vi "数字量输出自动检测_fast.vi"(11 "测试值":enum16{"0", "1"}(ring)) -> ()   [LabVIEW 2010]
uses:
  全局量/试验配置信息.vi
panel:
  in  "CAN端口":u16
  out "结束？":bool
  in  "同步_2":i32
  in  "同步_1":i32
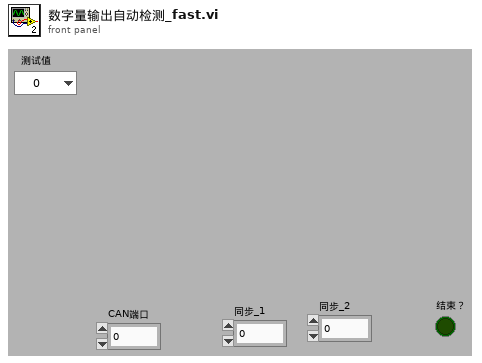
[diagram p1: front panel]
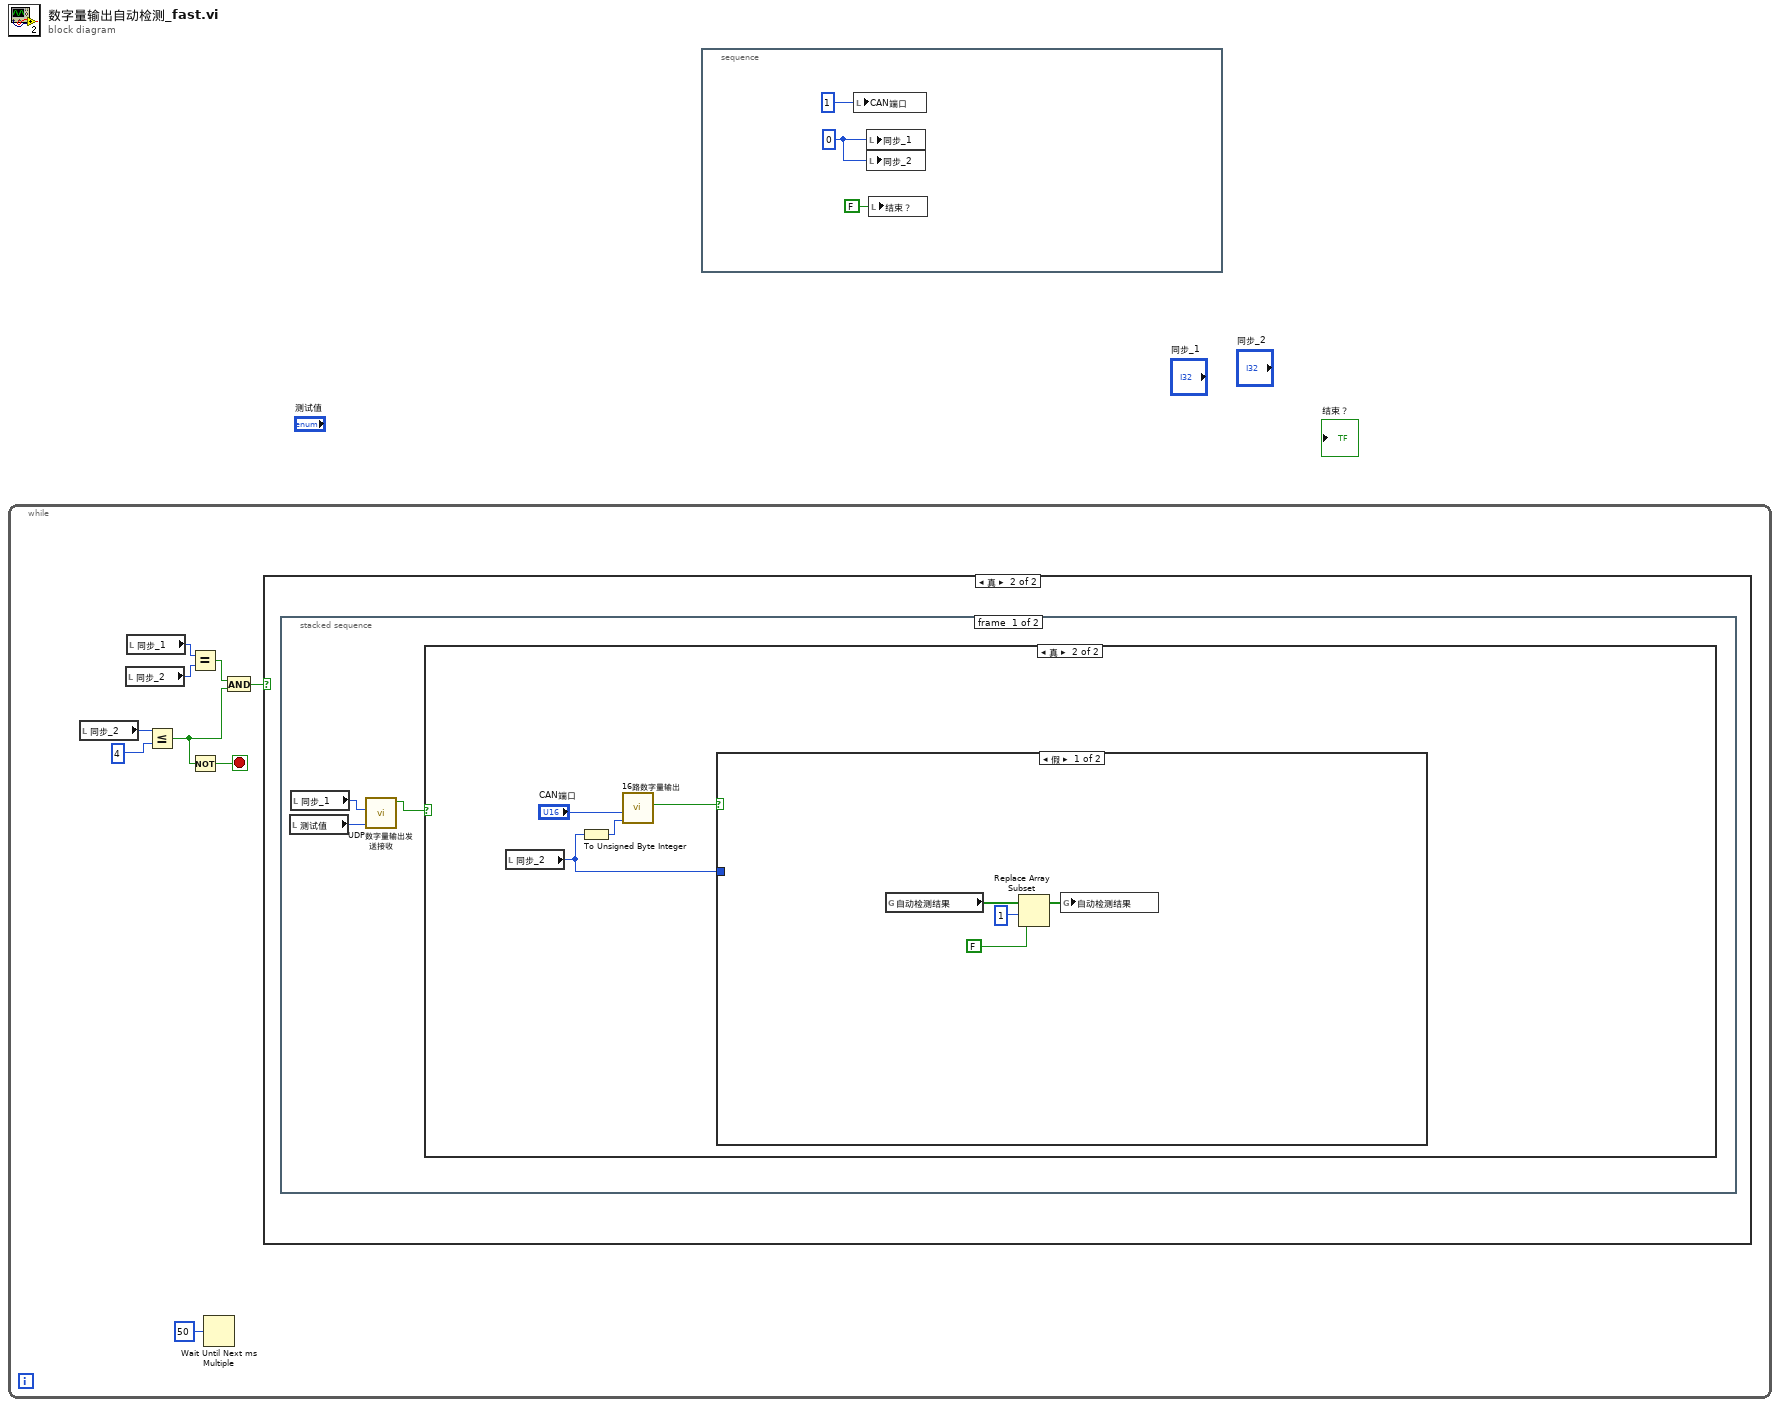
[diagram p0: block diagram]
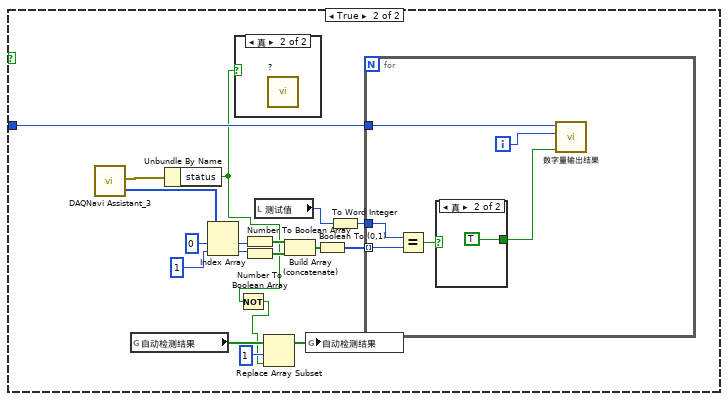
[diagram p4: hidden frame]
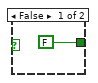
[diagram p6: hidden frame]
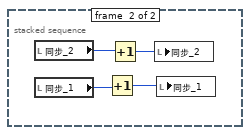
[diagram p7: hidden frame]
diagram:
  n1 = while {
    stop <- w4 stop-if-true
    n2 = local read "同步_2"() -> (w2:i32)
    n3 = local read "同步_2"() -> (w7:i32)
    n4 = local read "同步_1"() -> (w8:i32)
    n5 = Less Or Equal?(x=w2, y=4) -> (x <= y?=w3:bool)
    n6 = Equal?(x=w8, y=w7) -> (x = y?=w5:bool)
    n7 = Not(x=w3) -> (.not. x?=w4:bool)
    n8 = Wait Until Next ms Multiple(millisecond multiple=u32 50 ("毫秒倍数")) -> ()  [unwired: 1 out]
    n9 = And(x=w5, y=w3) -> (x .and. y?=w6:bool)
    n10 = case shown="真" w6 {
      frame False {
      }
      frame True {
        n11 = stacked-sequence {
          frame #0 {
            n12 = local read "测试值"() -> (w11:enum16{"0", "1"})
            n13 = local read "同步_1"() -> (w12:i32)
            n14 = call "UDP数字量输出发送接收.vi"("发送值"=w11, "第几组"=w12) -> ("正常_找到?"=w10:bool)  [unwired: 6 in, 3 out]
            n15 = case shown="真" w10 {
              frame False {
              }
              frame True {
                n16 = local read "同步_2"() -> (w16:i32)
                n17 = To Unsigned Byte Integer(number=w16) -> (unsigned 8bit integer=w14:u8)
                n18 = call "16路数字量输出.vi"("第几组数据"=w14, "CAN端口"="CAN端口") -> ("成功?"=w13:bool)  [unwired: 9 in]
                n19 = case shown="假" w13 {
                  tunnel: w16 -> [_ w38]
                  frame False {
                    n20 = global read "试验配置信息.vi" "自动检测结果"() -> (w18:bool[])
                    n21 = Replace Array Subset(array=w18, new element=FALSE ("新元素/子数组"), index=1 ("索引")) -> (w19:bool[])
                    n22 = global write "试验配置信息.vi" "自动检测结果"(w19) -> ()
                  }
                  frame True {
                    n23 = call "DAQNavi Assistant_3"() -> ("error out"=w30:errorcluster, "dataOut(U8Array)"=w31:u8[])  [unwired: 2 in, 16 out]
                    n24 = global read "试验配置信息.vi" "自动检测结果"() -> (w23:bool[])
                    n25 = Unbundle By Name(w30) -> ("status"=w21:bool)
                    n26 = Index Array(array=w31, index #1=0 ("索引"), index #2=1 ("索引")) -> (element #1=w26:u8, element #2=w29:u8)
                    n27 = case shown="真" w21 {
                      frame False {
                      }
                      frame True {
                        n28 = call "?"() -> ()  [unwired: 10 in, 2 out]
                      }
                    }
                    n29 = Not(x=w21) -> (.not. x?=w22:bool)
                    n30 = Number To Boolean Array(number=w26) -> (Boolean array=w36:bool[])
                    n31 = Number To Boolean Array(number=w29) -> (Boolean array=w37:bool[])
                    n32 = local read "测试值"() -> (w32:enum16{"0", "1"})
                    n33 = Replace Array Subset(array=w23, new element=w22, index=1 ("索引")) -> (w24:bool[])
                    n34 = Build Array (concatenate)(w36, w37) -> (w35:bool[])
                    n35 = global write "试验配置信息.vi" "自动检测结果"(w24) -> ()
                    n36 = Boolean To (0,1)(Boolean=w35) -> (0, 1=w34:i16[])
                    n37 = To Word Integer(number=w32) -> (16bit integer=w33:i16)
                    n38 = for {
                      tunnel: w34 -> [w42] mode=indexing
                      tunnel: w33 -> [w43]
                      tunnel: w38 -> [w41]
                      i -> [w40]
                      n39 = Equal?(x=w43, y=w42) -> (x = y?=w44:bool)
                      n40 = case shown="真" w44 {
                        tunnel: [FALSE TRUE] -> w39
                        frame False {
                        }
                        frame True {
                        }
                      }
                      n41 = call "数字量输出结果.vi"("合格?"=w39, "第几个"=w40, "第几组"=w41) -> ()  [unwired: 9 in]
                    }
                  }
                }
              }
            }
          }
          frame #1 {
            n42 = local read "同步_2"() -> (w50:i32)
            n43 = local read "同步_1"() -> (w48:i32)
            n44 = Increment(x=w48) -> (x+1=w47:i32)
            n45 = Increment(x=w50) -> (x+1=w49:i32)
            n46 = local write "同步_2"(w49) -> ()
            n47 = local write "同步_1"(w47) -> ()
          }
        }
      }
    }
  }
  n48 = stacked-sequence {
    frame #0 {
      w53 = 0 ("同步_1")
      n49 = local write "CAN端口"(u16 1 ("CAN端口")) -> ()
      n50 = local write "同步_1"(w53) -> ()
      n51 = local write "同步_2"(w53) -> ()
      n52 = local write "结束？"(FALSE ("结束？")) -> ()
    }
  }
